vi "Generate Quad Sample Array.vi"(0 "Rows to Init":i32=2000) -> (2 "TIME Array":dbl[](array[numeric]) format="%#.12f", 3 "PRESS Array":dbl[](array[numeric]) format="%#_10f", 4 "TEMP Array":dbl[](array[numeric]) format="%#_10f", 5 "DENS Array":dbl[](array[numeric]) format="%#_10f")   [LabVIEW 2023]
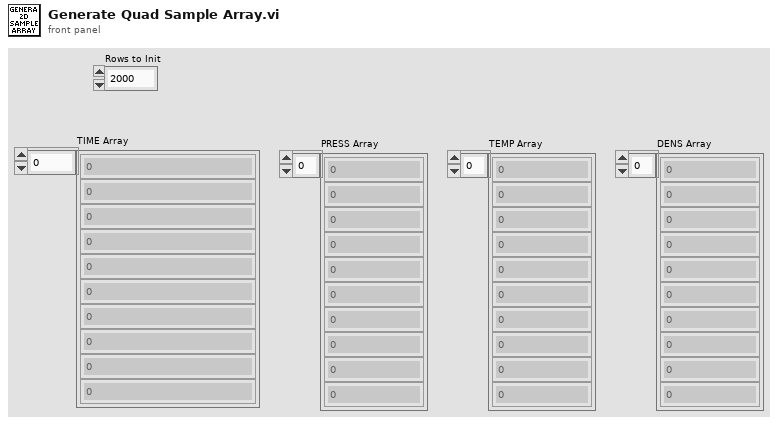
[diagram p1: front panel]
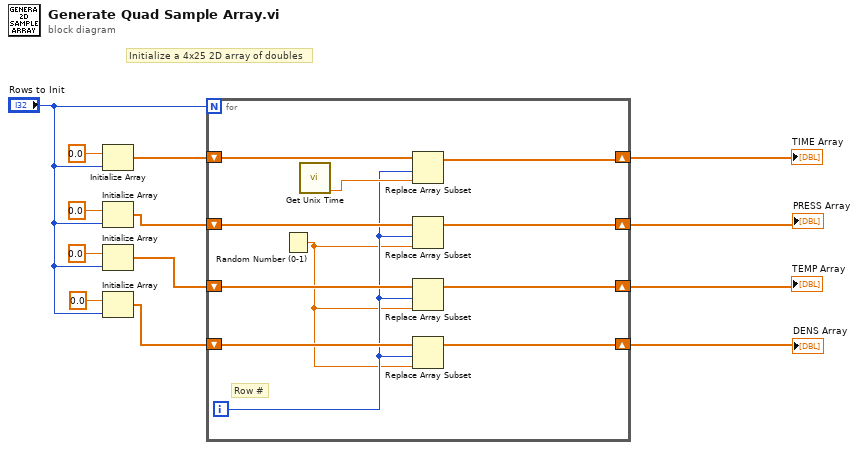
[diagram p0: block diagram]
diagram:
  # "Initialize a 4x25 2D array of doubles"
  n1 = Initialize Array(0.0, "Rows to Init") -> (w12:dbl[])
  n2 = Initialize Array(0.0, "Rows to Init") -> (w6:dbl[])
  n3 = Initialize Array(0.0, "Rows to Init") -> (w5:dbl[])
  n4 = Initialize Array(0.0, "Rows to Init") -> (w4:dbl[])
  n5 = for {
    N: "Rows to Init" -> [_]
    shift-right: [w23] -> w11
    shift-left: w12 -> [w24]
    shift-right: [w17] -> w3
    shift-left: w6 -> [w21]
    shift-right: [w16] -> w2
    shift-left: w5 -> [w20]
    shift-right: [w15] -> w1
    shift-left: w4 -> [w19]
    i -> [w18]
    # "Row #"
    n6 = Random Number (0-1)() -> (number: 0 to 1=w14:dbl)
    n7 = call "Get Unix Time.vi"() -> ("Unix Time"=w22:dbl)  [unwired: 10 in, 1 out]
    n8 = Replace Array Subset(array=w24, new element=w22, index=w18) -> (w23:dbl[])
    n9 = Replace Array Subset(array=w21, new element=w14, index=w18) -> (w17:dbl[])
    n10 = Replace Array Subset(array=w20, new element=w14, index=w18) -> (w16:dbl[])
    n11 = Replace Array Subset(array=w19, new element=w14, index=w18) -> (w15:dbl[])
  }
  "TIME Array" <- w11
  "PRESS Array" <- w3
  "TEMP Array" <- w2
  "DENS Array" <- w1
